vi "Image Draw.vi"(5 "Frame Properties (m)":T1, 7 "Reframed Position (m)":cluster{"x (m)":dbl, "y (m)":dbl, "z (m)":dbl} {"z (m)" format="%.1p"; "y (m)" format="%.1p"; "x (m)" format="%.1p"}, 8 "ih":i16, 9 "iw":i16, 10 "picture":picture) -> (2 "new picture":picture)   [LabVIEW 2017]
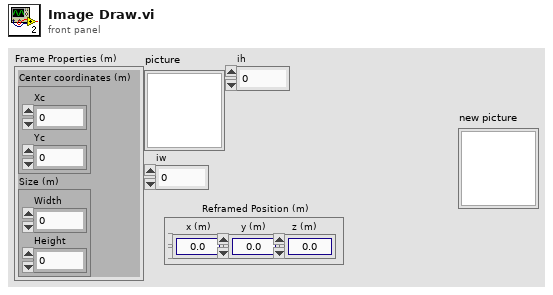
[diagram p1: front panel]
types:
  T1 = cluster{"Center coordinates (m)":cluster{"Xc":sgl, "Yc":sgl}, "Size (m)":cluster{"Width":sgl, "Height":sgl}}
  T2 = cluster{"left":i16, "top":i16, "right":i16, "bottom":i16}
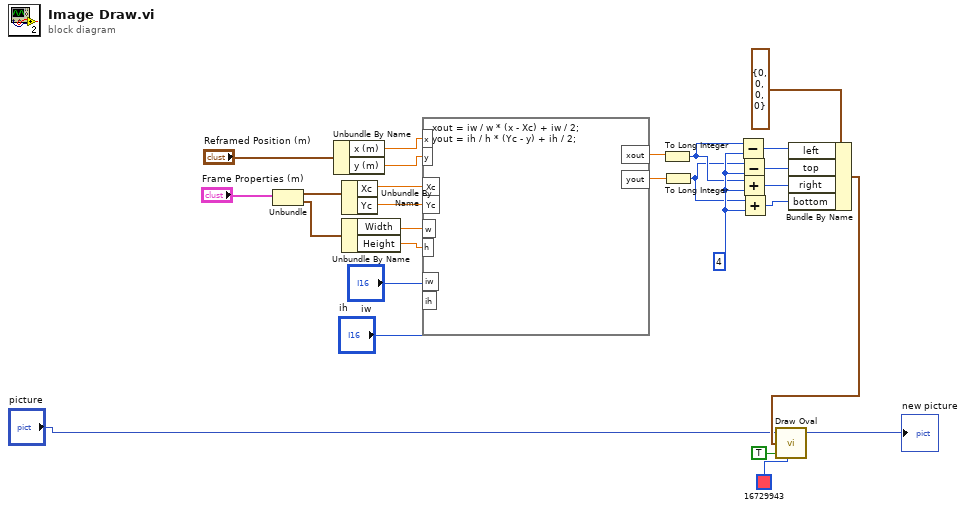
[diagram p0: block diagram]
diagram:
  w12 = 4
  n1 = Unbundle("Frame Properties (m)") -> ("Center coordinates (m)"=w25:cluster{"Xc":sgl, "Yc":sgl}, "Size (m)"=w24:cluster{"Width":sgl, "Height":sgl})
  n2 = Unbundle By Name("Reframed Position (m)") -> ("x (m)"=w23:dbl, "y (m)"=w22:dbl)
  n3 = Unbundle By Name(w25) -> ("Xc"=w21:sgl, "Yc"=w20:sgl)
  n4 = Unbundle By Name(w24) -> ("Width"=w19:sgl, "Height"=w18:sgl)
  n5 = formula code="xout = iw / w * (x - Xc) + iw / 2;\nyout = ih / h * (Yc - y) + ih / 2;"("x"=w23, "y"=w22, "Xc"=w21, "Yc"=w20, "w"=w19, "h"=w18, "iw"="iw", "ih"="ih") -> ("xout"=w16:dbl, "yout"=w17:dbl)
  n6 = To Long Integer(number=w16) -> (32bit integer=w11:i32)
  n7 = To Long Integer(number=w17) -> (32bit integer=w10:i32)
  n8 = Subtract(x=w11, y=w12) -> (x-y=w14:i32)
  n9 = Subtract(x=w10, y=w12) -> (x-y=w8:i32)
  n10 = Add(x=w11, y=w12) -> (x+y=w13:i32)
  n11 = Add(x=w10, y=w12) -> (x+y=w9:i32)
  n12 = Bundle By Name(cluster=T2 {"left"=0, "top"=0, "right"=0, "bottom"=0} ("rect"), "left"=w14, "top"=w8, "right"=w13, "bottom"=w9) -> (w7:T2)
  n13 = call <vilib>:"Draw Oval.vi"("picture"="picture", "rect"=w7, "fill?(F)"=TRUE, "color(black)"=u32 16729943) -> ("new picture"=→"new picture":picture)  [unwired: 5 in]
